vi "writeToXML.vi"(8 "error in (no error)":errorcluster, 10 "ClassLabel":string, 11 "Ephemeris in":refnum<class "Ephemeris.lvclass">) -> (0 "error out":errorcluster, 2 "XMLout":string, 3 "Ephemeris out":refnum<class "Ephemeris.lvclass">)   [LabVIEW 2022 SP3, in "TCSDataDefinitions.lvlib" / "TCSCommand.lvlib" / "TargetConfiguration.lvlib" / "Target.lvlib" / "Ephemeris.lvclass"]
uses:
  Ephemeris.lvclass
  Ephemeris.lvclass/Ephemeris.ctl
  Target/Target.lvclass
  <userlib>/Common/XML/XMLGenerator/XMLGenerator.lvclass
  <userlib>/Common/XML/XMLAttributeGenerator/XMLAttributeGenerator.lvclass
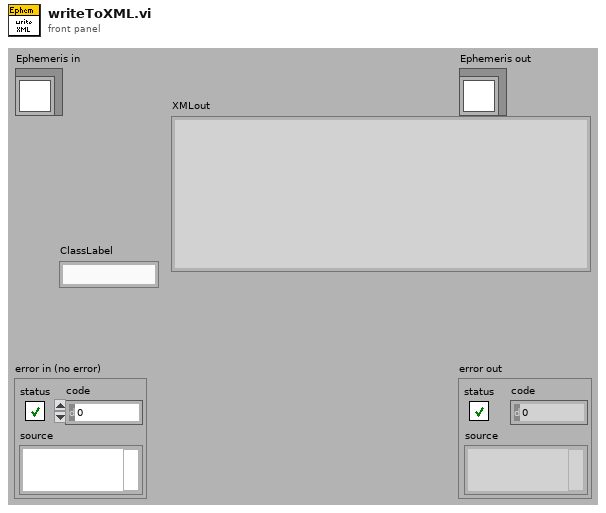
[diagram p1: front panel]
types:
  T1 = typedef "TCSDataDefinitions.lvlib/TCSCommand.lvlib/TargetConfiguration.lvlib/Target.lvlib/FixedTarget.lvlib/FrameValues.ctl" = enum16{"FK4", "FK5", "APPT", "GAPPT", "AZEL"}
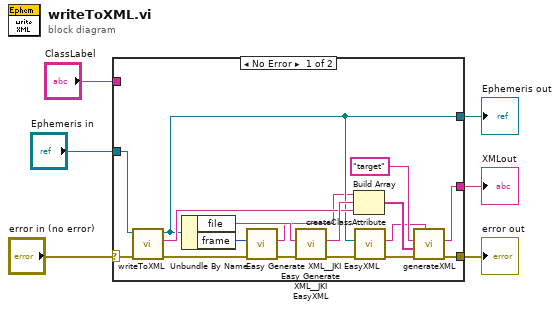
[diagram p0: block diagram]
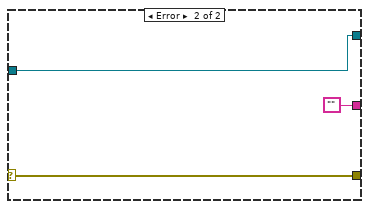
[diagram p2: hidden frame]
diagram:
  n1 = case shown="No Error" "error in (no error)" {
    selector: "error in (no error)" -> [w22 w26]
    tunnel: [w20 w26] -> w5
    tunnel: [w14 w25] -> w3
    tunnel: "Ephemeris in" -> [w23 w25]
    tunnel: [w16 ""] -> w2
    tunnel: "ClassLabel" -> [_ _]
    frame No Error {
      n2 = call-parent "writeToXML.vi"("error in (no error)"=w22, "Target in"=w23) -> ("error out"=w8:errorcluster, "XML out"=w15:string, "Target out"=w14:refnum<class "Ephemeris.lvclass">)  [unwired: 7 in]
      n3 = Unbundle By Name(w14) -> ("file"=w21:string, "frame"=w10:T1)
      n4 = call <vilib>:"Easy Generate XML__JKI EasyXML.vi"("error in (no error)"=w8, "LabVIEW Data"=w10) -> ("error out"=w7:errorcluster, "XML String"=w9:string)  [unwired: 8 in]
      n5 = call <vilib>:"Easy Generate XML__JKI EasyXML.vi"("error in (no error)"=w7, "LabVIEW Data"=w21) -> ("error out"=w13:errorcluster, "XML String"=w19:string)  [unwired: 8 in]
      n6 = Build Array(w9, w19, w15) -> (w18:string[])
      n7 = call <userlib>:"createClassAttribute.vi"("error in (no error)"=w13, "LVClass In"=w14) -> ("error out"=w12:errorcluster, "AttributeString"=w11:string)  [unwired: 7 in, 1 out]
      n8 = call <userlib>:"generateXML.vi"("attributeString"=w11, "error in"=w12, "childrenXML"=w18, "elementName"="target" ("Class Label")) -> ("error out"=w20:errorcluster, "XML out"=w16:string)  [unwired: 5 in, 1 out]
    }
    frame Error {
    }
  }
  "error out" <- w5
  "Ephemeris out" <- w3
  "XMLout" <- w2
